vi "Lin_Rohner_lab4B.vi"() -> ()   [LabVIEW 2019]
uses:
  <vilib>/Platform/TimedLoop/XDataNode/timing_clust.ctl
  <vilib>/Platform/TimedLoop/XDataNode/nitl_modes.ctl
  <vilib>/Platform/TimedLoop/XDataNode/wakeup.ctl
  <vilib>/Analysis/3filter.llb/Filter Passband Type.ctl
  <vilib>/DAQmx/write.llb/DAQmx Write (Analog DBL 1Chan 1Samp).vi
  <vilib>/DAQmx/read.llb/DAQmx Read (Analog DBL 1Chan 1Samp).vi
  <vilib>/DAQmx/create/channels.llb/DAQmx Create Channel (AO-Voltage-Basic).vi
  <vilib>/DAQmx/miscellaneous.llb/DAQmx Fill In Error Info.vi
  <vilib>/DAQmx/create/channels.llb/DAQmx Create Channel (AI-Voltage-Basic).vi
  <vilib>/platform/TimedLoop/XDataNode/XDataNode.xnode
  <vilib>/Platform/TimedLoop/XDataNode/XDNodeRunTimeDep.lvlib
  <vilib>/ptbypt/NI_PtbyPt.lvlib
  <vilib>/Analysis/NI_AALBase.lvlib
panel:
  out "Angular Position [deg]":dbl
  in  "B":dbl
  in  "K":dbl
  in  "Virtual Wall":bool
  in  "Velocity Filter":bool
  in  "Position Filter":bool
  out "Compensation Voltage":dbl
  out "Compensation Voltage":dbl(graph)
  out "Gravity Compesation":dbl
  out "Friction Compensation":dbl
  in  "Friction Compensation":bool
  out "Filtered Angular Velocity [rad/s]":dbl(graph)
  out "Filtered Angular Velocity [rad/s]":dbl
  in  "low cutoff freq:  Velocity":dbl=0.125 format="%0.3f"
  in  "Gravaty Compensation":bool
  out "Angular Position [rad]":dbl(graph)
  out "Angular Position [rad]":dbl
  out "Friction Compensation":dbl(graph)
  out "Gravity Compesation":dbl(graph)
  in  "low cutoff freq: Position":dbl=0.125 format="%0.3f"
  in  "stop":bool
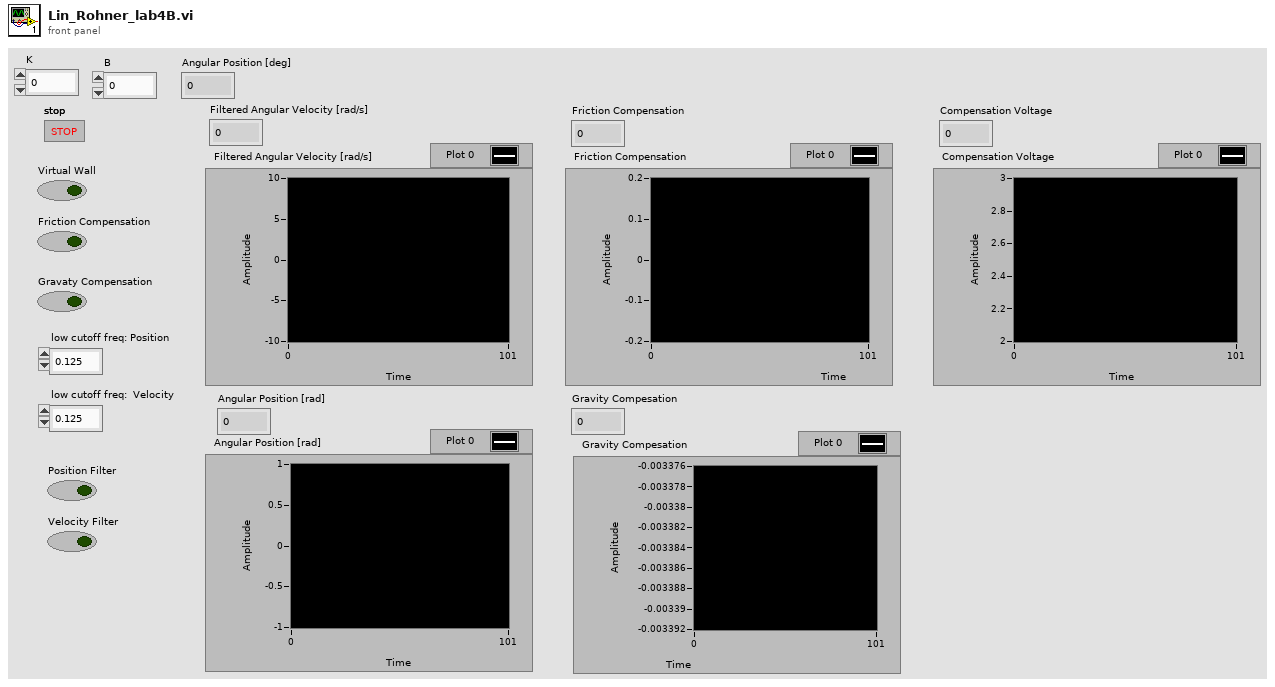
[diagram p1: front panel]
types:
  T1 = typedef "NI_AALBase.lvlib/Filter Passband Type.ctl" = enum32{"Lowpass", "Highpass", "Bandpass", "Bandstop"}
  T2 = typedef "XDNodeRunTimeDep.lvlib/timing_clust.ctl" = cluster{"Expected End [f-1]":u64, "Actual End [f-1]":u64, "Finished Late? [f-1]":bool, "Expected End [i-1]":u64, "Actual End [i-1]":u64, "Finished Late? [i-1]":bool, "Expected Start [i]":u64, "Actual Start [i]":u64, "Expected Start [f]":u64, "Actual Start [f]":u64, "Source Name":string, "Structure Name":string, "Period":i64, "Deadline":i64, "Offset":i64, "Start":i64, "Priority":i32, "Timeout":i32, "Mode":T3, "Wakeup Reason":T4, "Error":errorcluster, "Source Type":string, "Secondary Source Type":string, "Global End Time":u64, "Global Start Time":u64, "Frame Duration":u64, "Iteration Duration":u64, "Assigned CPU":i32, "I/O Scan Engine Mode":u32}
  T3 = typedef "XDNodeRunTimeDep.lvlib/nitl_modes.ctl" = enum32{"No Change", "Process missed periods, maintain original phase", "Discard missed periods, maintain original phase", "Process missed periods, ignore original phase", "Discard missed periods, ignore original phase"}
  T4 = typedef "XDNodeRunTimeDep.lvlib/wakeup.ctl" = enum32{"Normal", "Aborted", "Asynchronous wakeup", "Timing source error", "Timed loop error", "Timeout"}
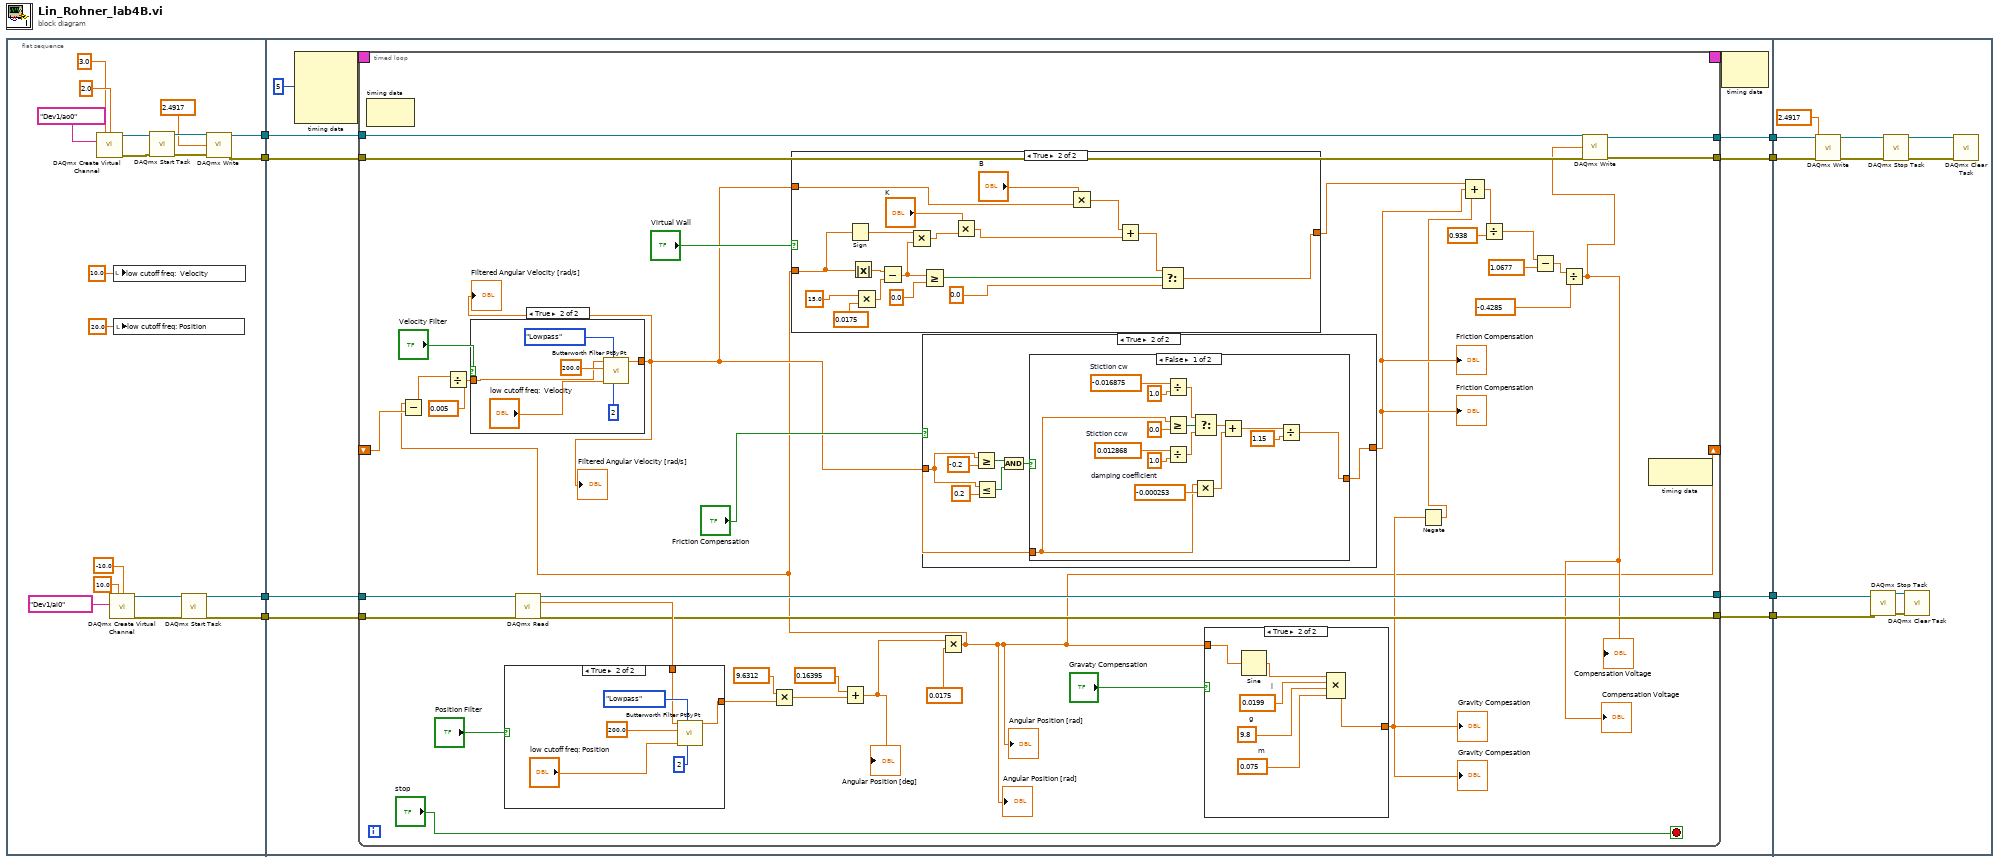
[diagram p0: block diagram]
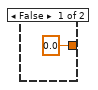
[diagram p2: hidden frame]
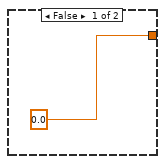
[diagram p5: hidden frame]
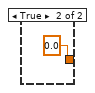
[diagram p6: hidden frame]
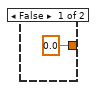
[diagram p7: hidden frame]
diagram:
  n1 = flat-sequence {
    tunnel: [w25] -> w8
    tunnel: [w24] -> w7
    tunnel: [w13] -> w6
    tunnel: [w12] -> w5
    tunnel: w8 -> [w35]
    tunnel: w7 -> [w34]
    tunnel: w6 -> [w33]
    tunnel: w5 -> [w32]
    tunnel: [w31] -> w4
    tunnel: [w30] -> w3
    tunnel: [w29] -> w2
    tunnel: [w28] -> w1
    tunnel: w4 -> [w150]
    tunnel: w3 -> [w149]
    tunnel: w2 -> [w148]
    tunnel: w1 -> [w147]
    frame #0 {
      n2 = call-poly <vilib>:"DAQmx Create Virtual Channel.vi"("maximum value"=3.0, "minimum value"=2.0, "physical channels"=tag "Dev1/ao0") -> ("task out"=w27:refnum<k21>, "error out"=w23:errorcluster)  [unwired: 11 in]
      n3 = call-poly <vilib>:"DAQmx Create Virtual Channel.vi"("maximum value"=10.0, "minimum value"=-10.0, "physical channels"=tag "Dev1/ai0") -> ("task out"=w14:refnum<k21>, "error out"=w15:errorcluster)  [unwired: 11 in]
      n4 = local write "low cutoff freq:  Velocity"(10.0 ("low cutoff freq:  Velocity")) -> ()
      n5 = local write "low cutoff freq: Position"(20.0 ("low cutoff freq: Position")) -> ()
      n6 = call <vilib>:"DAQmx Start Task.vi"("task/channels in"=w27, "error in"=w23) -> ("task out"=w26:refnum<k21>, "error out"=w22:errorcluster)  [unwired: 12 in]
      n7 = call <vilib>:"DAQmx Start Task.vi"("task/channels in"=w14, "error in"=w15) -> ("task out"=w13:refnum<k21>, "error out"=w12:errorcluster)  [unwired: 12 in]
      n8 = call-poly <vilib>:"DAQmx Write.vi"("task/channels in"=w26, "data"=2.4917, "error in"=w22) -> ("task out"=w25:refnum<k21>, "error out"=w24:errorcluster)  [unwired: 10 in, 1 out]
    }
    frame #1 {
      n9 = node-c288(i64 5 ("Period")) -> (w38:T2)  [unwired: 3 in]
      n10 = timed-loop {
        timing: w38 -> [_]
        timing-out: [_] -> w37
        tunnel: w35 -> [w71]
        tunnel: w34 -> [w70]
        tunnel: w33 -> [w69]
        tunnel: w32 -> [w68]
        tunnel: [w65] -> w31
        tunnel: [w64] -> w30
        tunnel: [w67] -> w29
        tunnel: [w66] -> w28
        shift-right: [w40] -> _
        shift-left: _ -> [w58]
        stop <- "stop" stop-if-true
        n11 = node-c288() -> ()  [unwired: 1 in, 1 out]
        n12 = call-poly <vilib>:"DAQmx Read.vi"("task/channels in"=w69, "error in"=w68) -> ("task out"=w67:refnum<k21>, "data"=w72:dbl, "error out"=w66:errorcluster)  [unwired: 11 in]
        n13 = case shown="True" "Position Filter" {
          tunnel: [w103 w106] -> w73
          tunnel: w72 -> [w103 w105]
          frame False {
          }
          frame True {
            n14 = call <vilib>:"Butterworth Filter PtByPt.vi"("order"=2, "filter type"=Filter_Passband_Type."Lowpass", "low cutoff freq: fl"="low cutoff freq: Position", "sampling freq: fs"=200.0, "x"=w105) -> ("Filtered x"=w106:dbl)  [unwired: 4 in, 1 out]
          }
        }
        n15 = Multiply(x=9.6312, y=w73) -> (x*y=w75:dbl)
        n16 = Add(x=0.16395, y=w75) -> (x+y=w39:dbl)
        "Angular Position [deg]" <- w39
        n17 = Multiply(x=w39, y=0.0175) -> (x*y=w40:dbl)
        "Angular Position [rad]" <- w40
        "Angular Position [rad]" <- w40
        n18 = Subtract(x=w40, y=w58) -> (x-y=w61:dbl)
        n19 = Divide(x=w61, y=0.005) -> (x/y=w59:dbl)
        n20 = case shown="True" "Velocity Filter" {
          tunnel: w59 -> [w96 w99]
          tunnel: [w96 w97] -> w41
          frame False {
          }
          frame True {
            n21 = call <vilib>:"Butterworth Filter PtByPt.vi"("order"=2, "filter type"=Filter_Passband_Type."Lowpass", "low cutoff freq: fl"="low cutoff freq:  Velocity", "sampling freq: fs"=200.0, "x"=w99) -> ("Filtered x"=w97:dbl)  [unwired: 4 in, 1 out]
          }
        }
        "Filtered Angular Velocity [rad/s]" <- w41
        "Filtered Angular Velocity [rad/s]" <- w41
        n22 = case shown="True" "Virtual Wall" {
          tunnel: w40 -> [_ w91]
          tunnel: w41 -> [_ w87]
          tunnel: [0.0 w83] -> w43
          frame False {
          }
          frame True {
            n23 = Sign(1:w91) -> (0:w90:dbl)
            n24 = Absolute Value(x=w91) -> (abs(x)=w94:dbl)
            n25 = Multiply(x=15.0 ("y"), y=0.0175) -> (x*y=w78:dbl)
            n26 = Subtract(x=w94, y=w78) -> (x-y=w89:dbl)
            n27 = Multiply(x=w90, y=w89) -> (x*y=w88:dbl)
            n28 = Greater Or Equal?(x=w89, y=0.0) -> (x >= y?=w92:bool)
            n29 = Multiply(x="K", y=w88) -> (x*y=w85:dbl)
            n30 = Multiply(x="B", y=w87) -> (x*y=w86:dbl)
            n31 = Add(x=w86, y=w85) -> (x+y=w84:dbl)
            n32 = Select(t=w84, s=w92, f=0.0) -> (s? t:f=w83:dbl)
          }
        }
        n33 = case shown="True" "Friction Compensation" {
          tunnel: [0.0 ("f") w112] -> w45
          tunnel: w41 -> [_ w111]
          frame False {
          }
          frame True {
            n34 = Greater Or Equal?(x=w111, y=-0.2) -> (x >= y?=w115:bool)
            n35 = Less Or Equal?(x=w111, y=0.2) -> (x <= y?=w114:bool)
            n36 = And(x=w115, y=w114) -> (x .and. y?=w113:bool)
            n37 = case shown="False" w113 {
              tunnel: [w119 0.0 ("y")] -> w112
              tunnel: w111 -> [w128 _]
              frame False {
                w130 = -0.000253  # damping coefficient
                w126 = 0.012868  # Stiction ccw
                w123 = -0.016875  # Stiction cw
                n38 = Divide(x=w123, y=1.0) -> (x/y=w122:dbl)
                n39 = Greater Or Equal?(x=w128, y=0.0) -> (x >= y?=w131:bool)
                n40 = Divide(x=w126, y=1.0) -> (x/y=w125:dbl)
                n41 = Multiply(x=w128, y=w130) -> (x*y=w129:dbl)
                n42 = Select(t=w122, s=w131, f=w125) -> (s? t:f=w127:dbl)
                n43 = Add(x=w127, y=w129) -> (x+y=w120:dbl)
                n44 = Divide(x=w120, y=1.15) -> (x/y=w119:dbl)
              }
              frame True {
              }
            }
          }
        }
        "Friction Compensation" <- w45
        "Friction Compensation" <- w45
        n45 = case shown="True" "Gravaty Compensation" {
          tunnel: [0.0 w136] -> w49
          tunnel: w40 -> [_ w135]
          frame False {
          }
          frame True {
            w137 = 0.075  # m
            w138 = 9.8  # g
            w139 = 0.0199  # l
            n46 = Sine(x=w135) -> (sin(x)=w140:dbl)
            n47 = Compound Arithmetic op=MULTIPLY(w140, w139, w138, w137) -> (w136:dbl)
          }
        }
        "Gravity Compesation" <- w49
        "Gravity Compesation" <- w49
        n48 = Negate(x=w49) -> (-x=w44:dbl)
        n49 = Compound Arithmetic op=ADD(w43, w45, w44) -> (w42:dbl)
        n50 = Divide(x=w42, y=0.938) -> (x/y=w54:dbl)
        n51 = Subtract(x=w54, y=1.0677) -> (x-y=w52:dbl)
        n52 = Divide(x=w52, y=-0.4285) -> (x/y=w50:dbl)
        "Compensation Voltage" <- w50
        "Compensation Voltage" <- w50
        n53 = call-poly <vilib>:"DAQmx Write.vi"("task/channels in"=w71, "data"=w50, "error in"=w70) -> ("task out"=w65:refnum<k21>, "error out"=w64:errorcluster)  [unwired: 10 in, 1 out]
        n54 = node-c288() -> ()  [unwired: 1 in, 1 out]
      }
      n55 = node-c288(w37) -> ()  [unwired: 1 out]
    }
    frame #2 {
      n56 = call-poly <vilib>:"DAQmx Write.vi"("task/channels in"=w150, "data"=2.4917, "error in"=w149) -> ("task out"=w157:refnum<k21>, "error out"=w154:errorcluster)  [unwired: 10 in, 1 out]
      n57 = call <vilib>:"DAQmx Stop Task.vi"("task/channels in"=w148, "error in"=w147) -> ("task out"=w151:refnum<k21>, "error out"=w152:errorcluster)  [unwired: 12 in]
      n58 = call <vilib>:"DAQmx Stop Task.vi"("task/channels in"=w157, "error in"=w154) -> ("task out"=w156:refnum<k21>, "error out"=w155:errorcluster)  [unwired: 12 in]
      n59 = call <vilib>:"DAQmx Clear Task.vi"("task in"=w151, "error in"=w152) -> ()  [unwired: 13 in, 1 out]
      n60 = call <vilib>:"DAQmx Clear Task.vi"("task in"=w156, "error in"=w155) -> ()  [unwired: 13 in, 1 out]
    }
  }
